vi "cntdwnmsg.vi"(10 "Boolean":bool, 11 "Numeric":i32) -> ()   [LabVIEW 2019]
panel:
  out "error out":errorcluster
  in  "error in (no error)":errorcluster
  out "OK":bool
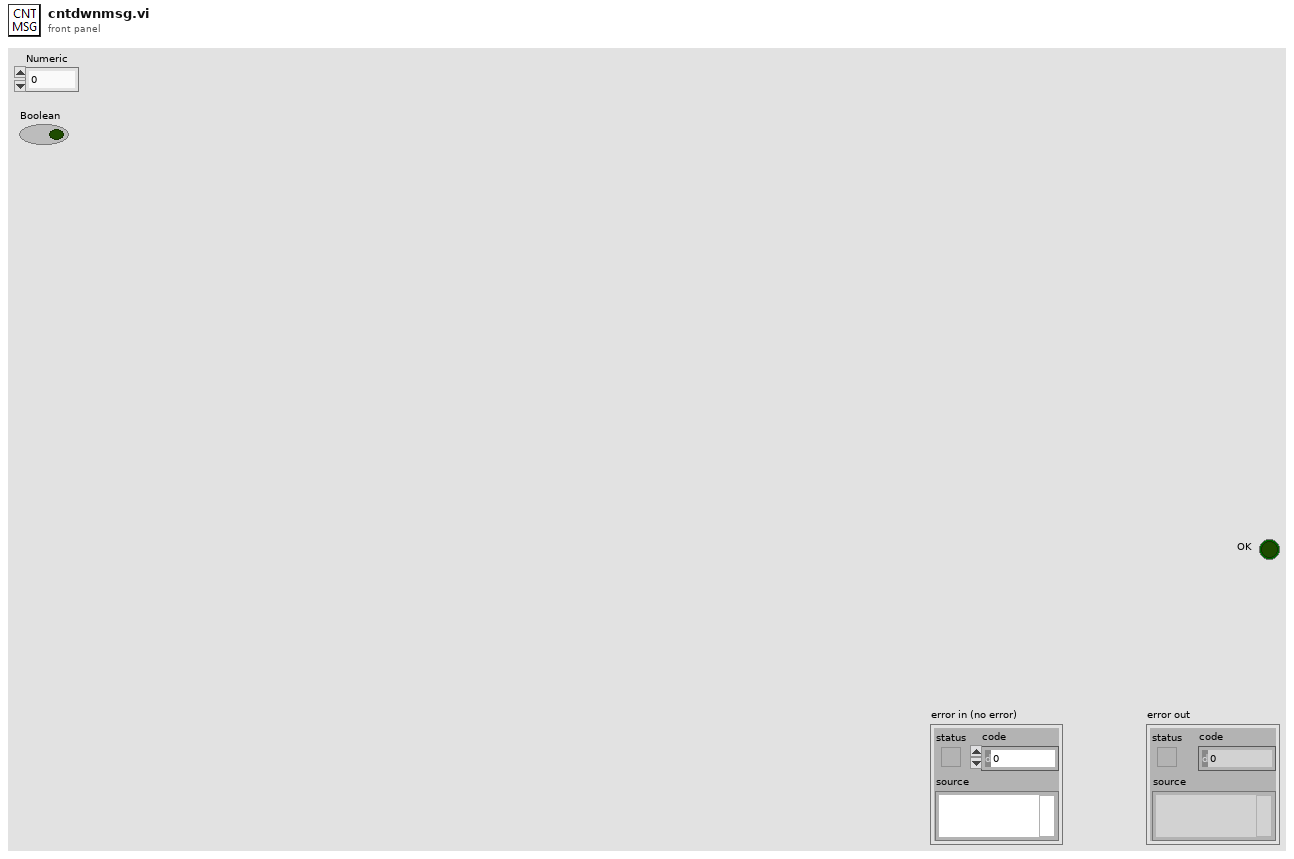
[diagram p1: front panel]
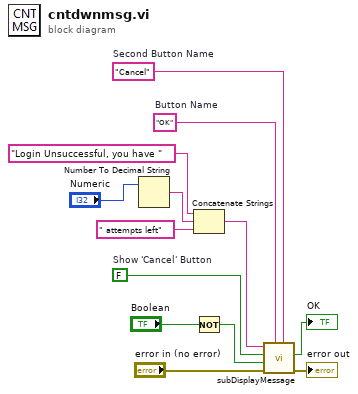
[diagram p0: block diagram]
diagram:
  w5 = "OK"  # Button Name
  w6 = "Cancel"  # Second Button Name
  w7 = FALSE  # Show 'Cancel' Button
  n1 = Number To Decimal String(number="Numeric") -> (decimal integer string=w12:string)  [unwired: 1 in]
  n2 = Concatenate Strings("Login Unsuccessful, you have " ("string"), w12, " attempts left" ("string")) -> (w1:string)
  n3 = Not(x="Boolean") -> (.not. x?=w2:bool)
  n4 = call <vilib>:"subDisplayMessage.vi"("Second Button Name"=w6, "Button Name"=w5, "error in (no error)"="error in (no error)", "Enable Message"=w2, "Show 'Cancel' Button"=w7, "Message to Display"=w1) -> ("error out"=→"error out":errorcluster, "OK?"=→"OK":bool)  [unwired: 4 in]
